vi "SP Read TDMS Graphics Properties.vi"(8 "error in (no error)":errorcluster, 10 "Group Name In":string, 11 "Source TDMS File In":refnum<k34>) -> (0 "error out":errorcluster, 1 "S Parameter Formatting":T1 {"Plots"."Ch 2"."Reference" format="%#.2g"; "Plots"."Ch 2"."Display Data" items=["Data", "Memory", "Data/Memory"]; "Plots"."Ch 2"."Format" items=["Log Mag", "Phase", "Expanded Phase", "Delay", "Smith", "Polar", "Lin Mag", "SWR", "Loss", "Real", "Imaginary"]; "Plots"."Ch 2"."Scale" min=0.001 step=1.0 format="%#.2g"; "Plots"."Ch 2"."Position" min=0.0 max=10.0; "Plots"."Ch 1"."Reference" format="%#.2g"; "Plots"."Ch 1"."Display Data" items=["Data", "Memory", "Data/Memory"]; "Plots"."Ch 1"."Format" items=["Log Mag", "Phase", "Expanded Phase", "Delay", "Smith", "Polar", "Lin Mag", "SWR", "Loss", "Real", "Imaginary"]; "Plots"."Ch 1"."Scale" min=0.001 step=1.0 format="%#.2g"; "Plots"."Ch 1"."Position" min=0.0 max=10.0}, 2 "Group Name Out":string, 3 "Source TDMS File Out":refnum<k34>)   [LabVIEW 2011]
uses:
  TypeDefs/SP Formatting.ctl
  TypeDefs/SP Plot Orientation.ctl
  TypeDefs/SP Plot.ctl
  TypeDefs/SP Trace Orientation.ctl
  TypeDefs/SP Display Trace Controls.ctl
  TypeDefs/SP Display Format.ctl
  TypeDefs/SP Display Data.ctl
  TypeDefs/SP Frequency Units.ctl
panel:
  # "Div"
  # "Div"
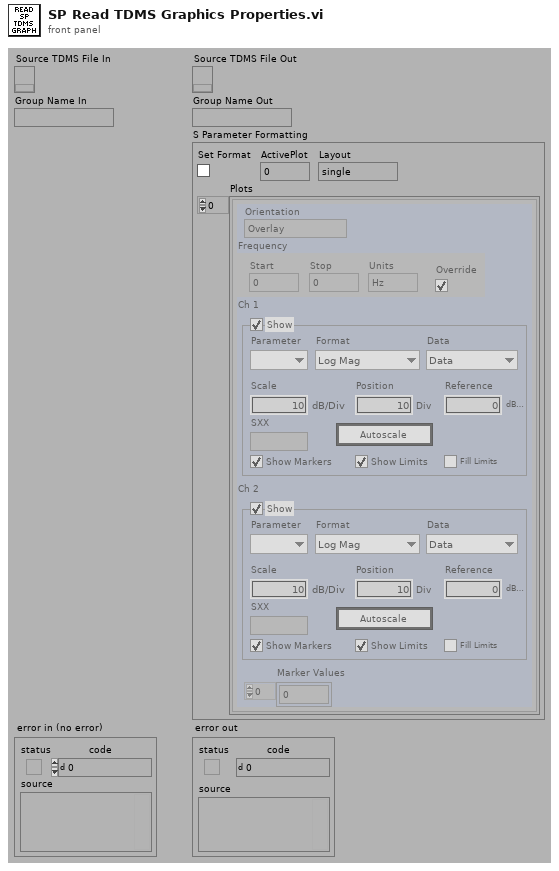
[diagram p1: front panel]
types:
  T1 = typedef "SP Formatting.ctl" = cluster{"Set Format":bool, "Layout":T2, "ActivePlot":i32, "Plots":T3[]}
  T2 = typedef "SP Plot Orientation.ctl" = enum32{"single", "dual", "quad"}
  T3 = typedef "SP Plot.ctl" = cluster{"Orientation":T4, "Ch 1":T5, "Ch 2":T5, "Frequency":cluster{"Start":dbl, "Stop":dbl, "Units":T8, "Override":bool}, "Marker Values":dbl[]}
  T4 = typedef "SP Trace Orientation.ctl" = enum32{"Overlay", "Split"}
  T5 = typedef "SP Display Trace Controls.ctl" = cluster{"Trace On":bool, "Measure":i32, "Format":T6, "Autoscale":bool, "Reference":dbl, "\nRefUnit":string, "Position":dbl, "Scale":dbl, "ScaleUnit":string, "LimitOn":bool, "LimitFill":bool, "Display Data":T7, "Show Markers":bool, "SXX":string}
  T6 = typedef "SP Display Format.ctl" = i32
  T7 = typedef "SP Display Data.ctl" = u16
  T8 = typedef "SP Frequency Units.ctl" = enum16{"Hz", "kHz", "MHz", "GHz", "Points"}
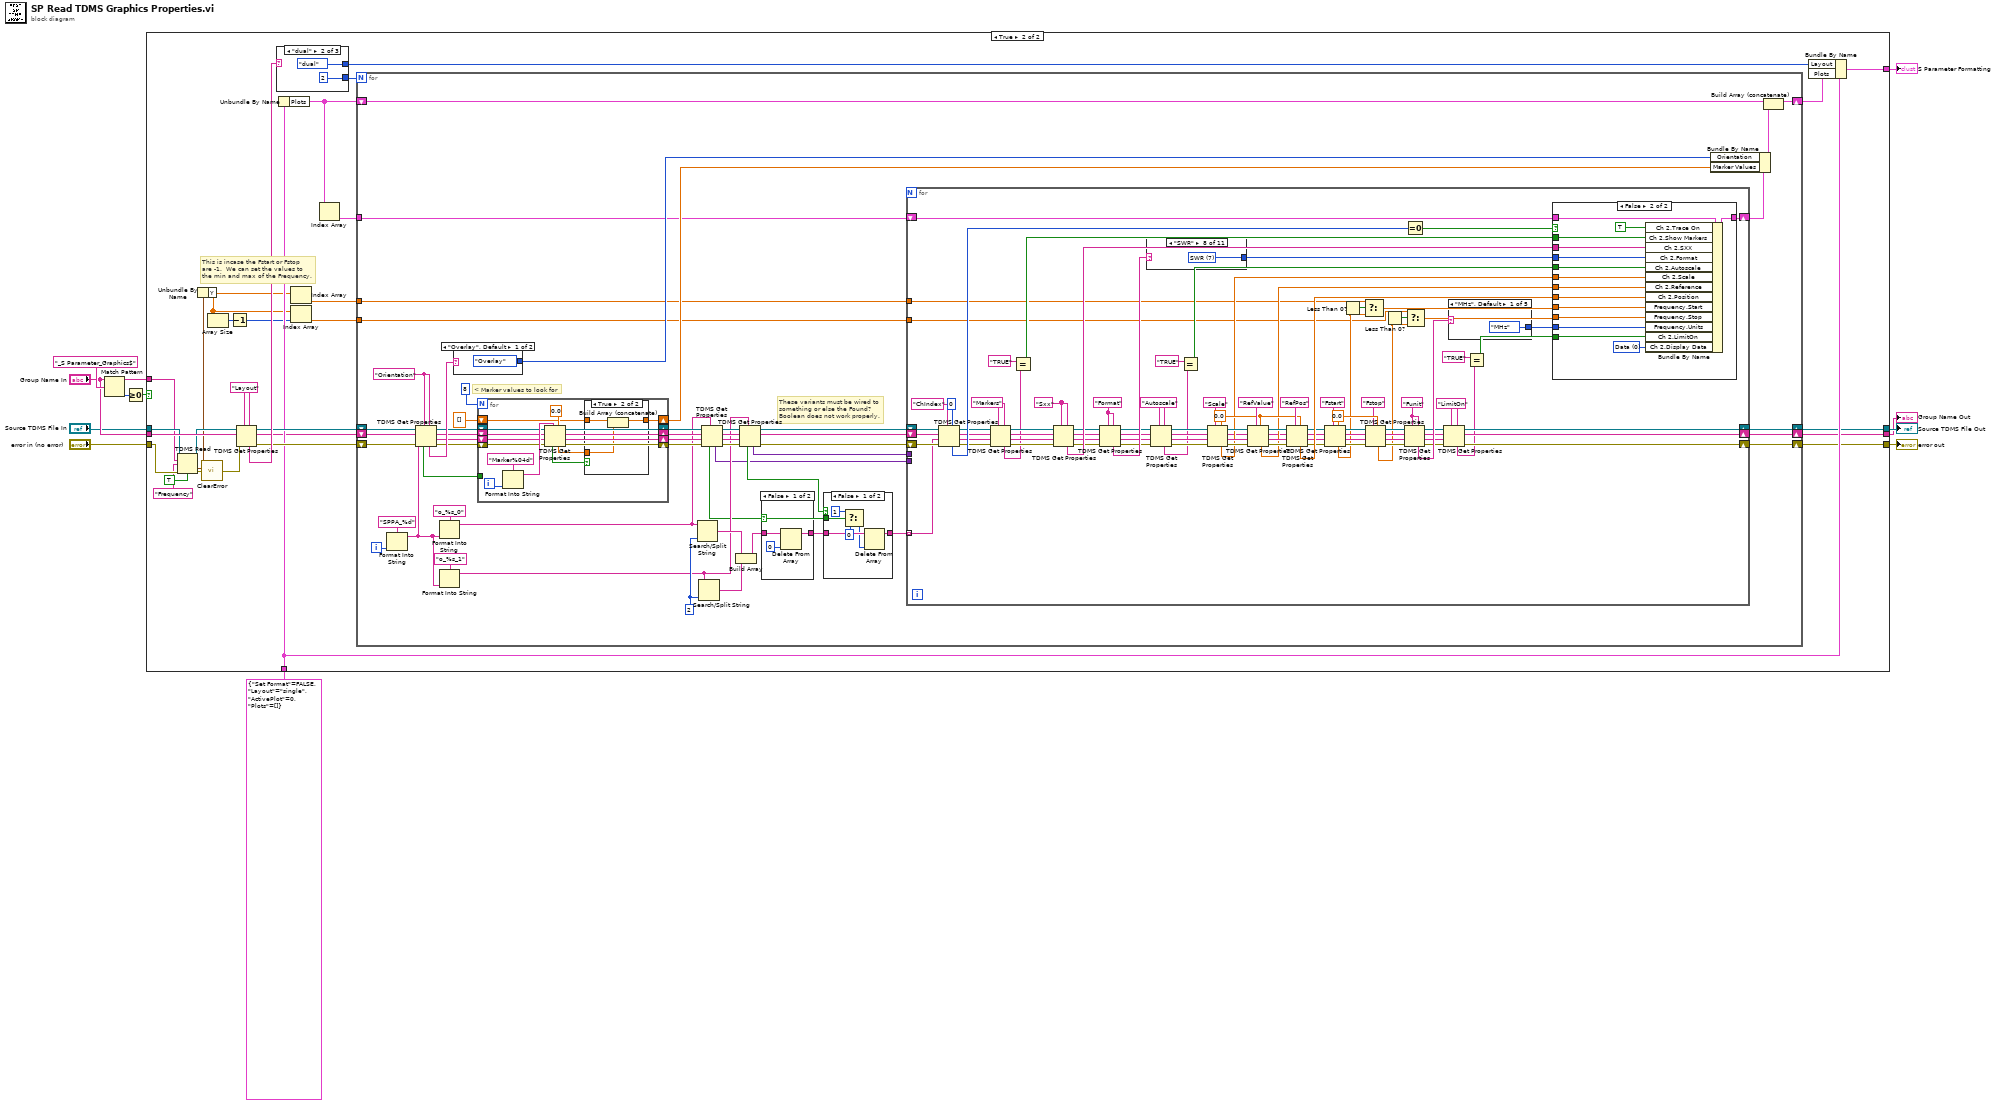
[diagram p0: block diagram]
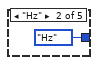
[diagram p3: hidden frame]
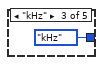
[diagram p4: hidden frame]
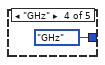
[diagram p5: hidden frame]
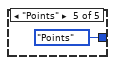
[diagram p6: hidden frame]
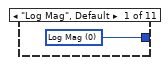
[diagram p7: hidden frame]
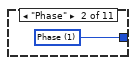
[diagram p8: hidden frame]
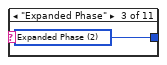
[diagram p9: hidden frame]
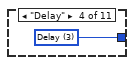
[diagram p10: hidden frame]
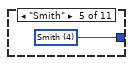
[diagram p11: hidden frame]
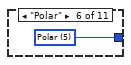
[diagram p12: hidden frame]
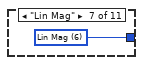
[diagram p13: hidden frame]
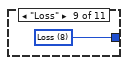
[diagram p14: hidden frame]
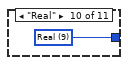
[diagram p15: hidden frame]
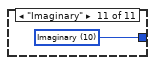
[diagram p16: hidden frame]
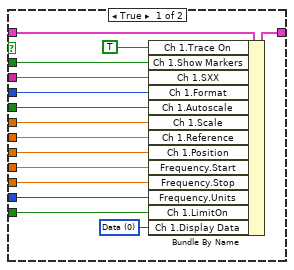
[diagram p17: hidden frame]
diagram:
  n1 = Match Pattern(string="Group Name In", regular expression="_S Parameter_Graphics$") -> (before substring=w1:string, offset past match=w9:i32)  [unwired: 3 out]
  n2 = Greater Or Equal To 0?(x=w9) -> (x >= 0?=w8:bool)
  n3 = case shown="True" w8 {
    tunnel: "error in (no error)" -> [w14 w30]
    tunnel: "Source TDMS File In" -> [w15 w29]
    tunnel: [w15 w37] -> w11
    tunnel: [w14 w36] -> w12
    tunnel: "Group Name In" -> [w13 w45]
    tunnel: T1 {"Set Format"=FALSE, "Layout"=enum."single", "ActivePlot"=0, "Plots"=[]} ("S Parameter Formatting") -> [_ w39]
    tunnel: [_ w33] -> w6
    tunnel: [w13 w32] -> w2
    tunnel: w1 -> [_ w26]
    frame False {
    }
    frame True {
      w21 = "Layout"
      # "This is incase the Fstart or Fstop\nare -1.  We can set the values to\nthe min and max of the Frequency."
      n4 = TDMS Read(0:w29, 5:w26, 7:"Frequency", 11:w30, 13:TRUE ("return channels in file order? (F)")) -> (4:w28:refnum<k34>, 10:w24:waveform(dbl), 15:w17:errorcluster)  [unwired: 3 in, 3 out]
      n5 = Unbundle By Name(w24) -> ("Y"=w22:dbl[])
      n6 = call <vilib>:"ClearError.vi"("error in (no error)"=w17) -> ("error out"=w27:errorcluster)
      n7 = Array Size(array=w22) -> (size(s)=w23:i32)
      n8 = Decrement(x=w23) -> (x-1=w18:i32)
      n9 = TDMS Get Properties(5:w21, 7:w21, 8:w27, 10:w45, 11:w28) -> (0:w41:errorcluster, 2:w31:string, 3:w40:refnum<k34>, 4:w44:string)  [unwired: 3 out]
      n10 = case shown="\"dual\"" w44 {
        tunnel: [SP_Plot_Orientation."single" ("Plot Orientation") SP_Plot_Orientation."dual" ("Plot Orientation") SP_Plot_Orientation."quad" ("Plot Orientation")] -> w43
        tunnel: [1 2 4] -> w42
        frame "single", Default {
        }
        frame "dual" {
        }
        frame "quad" {
        }
      }
      n11 = Unbundle By Name(w39) -> ("Plots"=w35:T3[])
      n12 = Index Array(array=w22) -> (element=w20:dbl)  [unwired: 1 in]
      n13 = Index Array(array=w22, index=w18) -> (element=w19:dbl)
      n14 = Index Array(array=w35) -> (element=w34:T3)  [unwired: 1 in]
      n15 = for {
        N: w42 -> [_]
        shift-right: [w93] -> w38
        shift-left: w35 -> [w94]
        shift-right: [w62] -> w37
        shift-left: w40 -> [w53]
        shift-right: [w63] -> w36
        shift-left: w41 -> [w97]
        tunnel: w34 -> [w65]
        shift-right: [w57] -> w32
        shift-left: w31 -> [w52]
        tunnel: w20 -> [w47]
        tunnel: w19 -> [w46]
        i -> [w95]
        w73 = 2 ("offset (0)")
        w89 = "Orientation"
        # "These variants must be wired to\nsomething or else the Found?\nBoolean does not work properly."
        # "< Marker values to look for"
        n16 = Format Into String(format string="SPPA_%d", w95) -> (resulting string=w78:string)  [unwired: 2 in, 1 out]
        n17 = TDMS Get Properties(5:w89, 7:w89, 8:w97, 9:w78, 10:w52, 11:w53) -> (0:w84:errorcluster, 1:w79:string, 2:w61:string, 3:w85:refnum<k34>, 4:w91:string, 6:w54:bool)
        n18 = Format Into String(format string="o_%s_0", w78) -> (resulting string=w56:string)  [unwired: 2 in, 1 out]
        n19 = Format Into String(format string="o_%s_1", w78) -> (resulting string=w55:string)  [unwired: 2 in, 1 out]
        n20 = case shown="\"Overlay\", Default" w91 {
          tunnel: [SP_Trace_Orientation."Overlay" ("Orientation") SP_Trace_Orientation."Split" ("Orientation")] -> w90
          frame "Overlay", Default {
          }
          frame "Split" {
          }
        }
        n21 = for {
          N: 8 -> [_]
          shift-right: [w258] -> w86
          shift-left: dbl[] [] ("Marker Values") -> [w260]
          shift-right: [w255] -> w83
          shift-left: w85 -> [w257]
          shift-right: [w254] -> w82
          shift-left: w84 -> [w256]
          shift-right: [w250] -> w60
          shift-left: w61 -> [w251]
          shift-right: [w252] -> w77
          shift-left: w79 -> [w253]
          tunnel: w54 -> [_]
          i -> [w264]
          n22 = Format Into String(format string="Marker%04d", w264) -> (resulting string=w263:string)  [unwired: 2 in, 1 out]
          n23 = TDMS Get Properties(5:0.0, 7:w263, 8:w256, 9:w253, 10:w251, 11:w257) -> (0:w254:errorcluster, 1:w252:string, 2:w250:string, 3:w255:refnum<k34>, 4:w259:dbl, 6:w261:bool)
          n24 = case shown="True" w261 {
            tunnel: w260 -> [w266 w269]
            tunnel: w259 -> [_ w268]
            tunnel: [w266 w267] -> w258
            frame False {
            }
            frame True {
              n25 = Build Array (concatenate)(w269, w268) -> (w267:dbl[])
            }
          }
        }
        n26 = Search/Split String(string=w56, offset (0)=w73) -> (match + rest of string=w71:string)  [unwired: 3 out]
        n27 = Search/Split String(string=w55, offset (0)=w73) -> (match + rest of string=w72:string)  [unwired: 3 out]
        n28 = TDMS Get Properties(7:w56, 8:w82, 9:w77, 10:w60, 11:w83) -> (0:w74:errorcluster, 1:w75:string, 2:w59:string, 3:w76:refnum<k34>, 4:w49:variant, 6:w50:bool)  [unwired: 1 out]
        n29 = Build Array(w71, w72) -> (w70:string[])
        n30 = TDMS Get Properties(7:w55, 8:w74, 9:w75, 10:w59, 11:w76) -> (0:w68:errorcluster, 2:w58:string, 3:w67:refnum<k34>, 4:w48:variant, 6:w51:bool)  [unwired: 2 out]
        n31 = case shown="False" w50 {
          tunnel: w70 -> [w248 w249]
          tunnel: [w247 w249] -> w69
          frame False {
            n32 = Delete From Array(array=w248, index=0) -> (array with subset deleted=w247:string[])  [unwired: 1 in, 1 out]
          }
          frame True {
          }
        }
        n33 = case shown="False" w51 {
          tunnel: w69 -> [w244 w245]
          tunnel: [w243 w245] -> w66
          tunnel: w50 -> [w242 _]
          frame False {
            n34 = Select(t=1 ("index"), s=w242, f=0 ("index")) -> (s? t:f=w239:i32)
            n35 = Delete From Array(array=w244, index=w239) -> (array with subset deleted=w243:string[])  [unwired: 1 in, 1 out]
          }
          frame True {
          }
        }
        n36 = for {
          shift-right: [w131] -> w63
          shift-left: w68 -> [w192]
          shift-right: [w132] -> w62
          shift-left: w67 -> [w191]
          tunnel: w66 -> [w183] mode=indexing
          shift-right: [w186] -> w64
          shift-left: w65 -> [w182]
          shift-right: [w118] -> w57
          shift-left: w58 -> [w130]
          tunnel: w49 -> [_]
          tunnel: w48 -> [_]
          tunnel: w47 -> [w99]
          tunnel: w46 -> [w98]
          w117 = "LimitOn"
          w150 = 0.0
          w138 = "Funit"
          w154 = 0.0
          w116 = "Autoscale"
          w172 = "Format"
          w177 = "Sxx"
          w115 = "Markers"
          n37 = TDMS Get Properties(5:0, 7:"ChIndex", 8:w192, 9:w183, 10:w130, 11:w191) -> (0:w184:errorcluster, 1:w179:string, 2:w129:string, 3:w185:refnum<k34>, 4:w188:i32)  [unwired: 1 out]
          n38 = TDMS Get Properties(5:w115, 7:w115, 8:w184, 9:w179, 10:w129, 11:w185) -> (0:w180:errorcluster, 1:w178:string, 2:w128:string, 3:w181:refnum<k34>, 4:w110:string)  [unwired: 1 out]
          n39 = Equal?(x="TRUE" ("y"), y=w110) -> (x = y?=w109:bool)
          n40 = TDMS Get Properties(5:w177, 7:w177, 8:w180, 9:w178, 10:w128, 11:w181) -> (0:w174:errorcluster, 1:w173:string, 2:w127:string, 3:w175:refnum<k34>, 4:w176:string)  [unwired: 1 out]
          n41 = TDMS Get Properties(5:w172, 7:w172, 8:w174, 9:w173, 10:w127, 11:w175) -> (0:w168:errorcluster, 1:w162:string, 2:w126:string, 3:w169:refnum<k34>, 4:w171:string)  [unwired: 1 out]
          n42 = case shown="\"SWR\"" w171 {
            tunnel: [w198 w199 w200 w201 w202 w203 w204 w205 w206 w207 w208] -> w170
            frame "Log Mag", Default {
              w198 = T6 0 items=["Log Mag", "Phase", "Expanded Phase", "Delay", "Smith", "Polar", "Lin Mag", "SWR", "Loss", "Real", "Imaginary"] ("Ch 1.Format")
            }
            frame "Phase" {
              w199 = T6 1 items=["Log Mag", "Phase", "Expanded Phase", "Delay", "Smith", "Polar", "Lin Mag", "SWR", "Loss", "Real", "Imaginary"] ("Ch 1.Format")
            }
            frame "Expanded Phase" {
              w200 = T6 2 items=["Log Mag", "Phase", "Expanded Phase", "Delay", "Smith", "Polar", "Lin Mag", "SWR", "Loss", "Real", "Imaginary"] ("Ch 1.Format")
            }
            frame "Delay" {
              w201 = T6 3 items=["Log Mag", "Phase", "Expanded Phase", "Delay", "Smith", "Polar", "Lin Mag", "SWR", "Loss", "Real", "Imaginary"] ("Ch 1.Format")
            }
            frame "Smith" {
              w202 = T6 4 items=["Log Mag", "Phase", "Expanded Phase", "Delay", "Smith", "Polar", "Lin Mag", "SWR", "Loss", "Real", "Imaginary"] ("Ch 1.Format")
            }
            frame "Polar" {
              w203 = T6 5 items=["Log Mag", "Phase", "Expanded Phase", "Delay", "Smith", "Polar", "Lin Mag", "SWR", "Loss", "Real", "Imaginary"] ("Ch 1.Format")
            }
            frame "Lin Mag" {
              w204 = T6 6 items=["Log Mag", "Phase", "Expanded Phase", "Delay", "Smith", "Polar", "Lin Mag", "SWR", "Loss", "Real", "Imaginary"] ("Ch 1.Format")
            }
            frame "SWR" {
              w205 = T6 7 items=["Log Mag", "Phase", "Expanded Phase", "Delay", "Smith", "Polar", "Lin Mag", "SWR", "Loss", "Real", "Imaginary"] ("Ch 1.Format")
            }
            frame "Loss" {
              w206 = T6 8 items=["Log Mag", "Phase", "Expanded Phase", "Delay", "Smith", "Polar", "Lin Mag", "SWR", "Loss", "Real", "Imaginary"] ("Ch 1.Format")
            }
            frame "Real" {
              w207 = T6 9 items=["Log Mag", "Phase", "Expanded Phase", "Delay", "Smith", "Polar", "Lin Mag", "SWR", "Loss", "Real", "Imaginary"] ("Ch 1.Format")
            }
            frame "Imaginary" {
              w208 = T6 10 items=["Log Mag", "Phase", "Expanded Phase", "Delay", "Smith", "Polar", "Lin Mag", "SWR", "Loss", "Real", "Imaginary"] ("Ch 1.Format")
            }
          }
          n43 = TDMS Get Properties(5:w116, 7:w116, 8:w168, 9:w162, 10:w126, 11:w169) -> (0:w158:errorcluster, 1:w161:string, 2:w125:string, 3:w164:refnum<k34>, 4:w113:string)  [unwired: 1 out]
          n44 = Equal?(x="TRUE" ("y"), y=w113) -> (x = y?=w114:bool)
          n45 = TDMS Get Properties(5:w154, 7:"Scale", 8:w158, 9:w161, 10:w125, 11:w164) -> (0:w157:errorcluster, 1:w160:string, 2:w124:string, 3:w163:refnum<k34>, 4:w153:dbl)  [unwired: 1 out]
          n46 = TDMS Get Properties(5:w154, 7:"RefValue", 8:w157, 9:w160, 10:w124, 11:w163) -> (0:w156:errorcluster, 1:w159:string, 2:w123:string, 3:w155:refnum<k34>, 4:w152:dbl)  [unwired: 1 out]
          n47 = TDMS Get Properties(5:w154, 7:"RefPos", 8:w156, 9:w159, 10:w123, 11:w155) -> (0:w140:errorcluster, 1:w139:string, 2:w122:string, 3:w141:refnum<k34>, 4:w151:dbl)  [unwired: 1 out]
          n48 = TDMS Get Properties(5:w150, 7:"Fstart", 8:w140, 9:w139, 10:w122, 11:w141) -> (0:w147:errorcluster, 1:w145:string, 2:w121:string, 3:w144:refnum<k34>, 4:w103:dbl)  [unwired: 1 out]
          n49 = Less Than 0?(x=w103) -> (x < 0?=w105:bool)
          n50 = Select(t=w99, s=w105, f=w103) -> (s? t:f=w100:dbl)
          n51 = TDMS Get Properties(5:w150, 7:"Fstop", 8:w147, 9:w145, 10:w121, 11:w144) -> (0:w148:errorcluster, 1:w146:string, 2:w120:string, 3:w149:refnum<k34>, 4:w102:dbl)  [unwired: 1 out]
          n52 = Less Than 0?(x=w102) -> (x < 0?=w104:bool)
          n53 = TDMS Get Properties(5:w138, 7:w138, 8:w148, 9:w146, 10:w120, 11:w149) -> (0:w134:errorcluster, 1:w133:string, 2:w119:string, 3:w135:refnum<k34>, 4:w137:string)  [unwired: 1 out]
          n54 = Equal To 0?(x=w188) -> (x = 0?=w187:bool)
          n55 = Select(t=w98, s=w104, f=w102) -> (s? t:f=w101:dbl)
          n56 = TDMS Get Properties(5:w117, 7:w117, 8:w134, 9:w133, 10:w119, 11:w135) -> (0:w131:errorcluster, 2:w118:string, 3:w132:refnum<k34>, 4:w107:string)  [unwired: 2 out]
          n57 = case shown="\"MHz\", Default" w137 {
            tunnel: [SP_Frequency_Units."MHz" ("Funit") SP_Frequency_Units."Hz" ("Funit") SP_Frequency_Units."kHz" ("Funit") SP_Frequency_Units."GHz" ("Funit") SP_Frequency_Units."Points" ("Funit")] -> w136
            frame "MHz", Default {
            }
            frame "Hz" {
            }
            frame "kHz" {
            }
            frame "GHz" {
            }
            frame "Points" {
            }
          }
          n58 = Equal?(x="TRUE" ("y"), y=w107) -> (x = y?=w106:bool)
          n59 = case shown="False" w187 {
            tunnel: w182 -> [w223 w238]
            tunnel: [w222 w237] -> w186
            tunnel: w109 -> [w220 w235]
            tunnel: w176 -> [w219 w234]
            tunnel: w170 -> [w218 w233]
            tunnel: w114 -> [w217 w232]
            tunnel: w153 -> [w216 w231]
            tunnel: w152 -> [w215 w230]
            tunnel: w151 -> [w214 w229]
            tunnel: w100 -> [w213 w228]
            tunnel: w101 -> [w212 w227]
            tunnel: w136 -> [w211 w226]
            tunnel: w106 -> [w210 w225]
            frame True {
              w209 = T7 0 items=["Data", "Memory", "Data/Memory"] ("Ch 1.Display Data")
              n60 = Bundle By Name(cluster=w223, "Ch 1.Trace On"=TRUE, "Ch 1.Show Markers"=w220, "Ch 1.SXX"=w219, "Ch 1.Format"=w218, "Ch 1.Autoscale"=w217, "Ch 1.Scale"=w216, "Ch 1.Reference"=w215, "Ch 1.Position"=w214, "Frequency.Start"=w213, "Frequency.Stop"=w212, "Frequency.Units"=w211, "Ch 1.LimitOn"=w210, "Ch 1.Display Data"=w209) -> (w222:T3)
            }
            frame False {
              w224 = T7 0 items=["Data", "Memory", "Data/Memory"] ("Ch 1.Display Data")
              n61 = Bundle By Name(cluster=w238, "Ch 2.Trace On"=TRUE, "Ch 2.Show Markers"=w235, "Ch 2.SXX"=w234, "Ch 2.Format"=w233, "Ch 2.Autoscale"=w232, "Ch 2.Scale"=w231, "Ch 2.Reference"=w230, "Ch 2.Position"=w229, "Frequency.Start"=w228, "Frequency.Stop"=w227, "Frequency.Units"=w226, "Ch 2.LimitOn"=w225, "Ch 2.Display Data"=w224) -> (w237:T3)
            }
          }
        }
        n62 = Bundle By Name(cluster=w64, "Orientation"=w90, "Marker Values"=w86) -> (w92:T3)
        n63 = Build Array (concatenate)(w94, w92) -> (w93:T3[])
      }
      n64 = Bundle By Name(cluster=w39, "Layout"=w43, "Plots"=w38) -> (w33:T1)
    }
  }
  "error out" <- w12
  "S Parameter Formatting" <- w6
  "Source TDMS File Out" <- w11
  "Group Name Out" <- w2
